vi "unwrap_phase_map_edge_detect_float.vi"(11 "u8_ar_dist_phasemap":dbl[][](array[numeric])=array1050x1050[1102500 elements]) -> (2 "df_ar_unwrapped_px_ar":dbl[][](array[numeric]), 3 "Refnum out":T3(plugin-control))   [LabVIEW 2011]
doc: "Takes a the warpped phase mapped as a pixel array and unwrappes it. Optional normalization from 0 to 255 for the pixel array output"
uses:
  <vilib>/vision/Measure.llb/Edge Options.ctl
  <vilib>/vision/Measure.llb/Edge Polarity.ctl
  global_vars.vi
  <vilib>/vision/NI_Vision_Development_Module.lvlib
panel:
  out "norm part":i16[](graph)
  out "unwrapped":dbl[](graph)
  out "norm factor":dbl
  out "offset":i16
  out "Intensity Graph 2":dbl[][](graph)
  out "Intensity Graph":dbl[][](graph)
  out "normalized array":u8[](array[numeric])
  out "normalized":u8[](graph)
  in  "Edge Options 3":T1={"Edge Polarity"=0, "Kernel Size"=3, "Width"=1, "Minimum Edge Strength"=250.0, "Interpolation Type"=enum."Bilinear Fixed", "Data Processing Method"=enum."Median"} {"Edge Polarity" items=["All Edges", "Rising Edges", "Falling Edges"]; "Minimum Edge Strength" format="%.2f"; "Width" step=2; "Kernel Size" step=2}
  out "start and end":i32[](array[numeric])
  out "edges":i16[](array[numeric])
  in  "stop":bool
  out "input":i16[](graph)
  in  "Edge Options 2":T1={"Edge Polarity"=0, "Kernel Size"=3, "Width"=1, "Minimum Edge Strength"=250.0, "Interpolation Type"=enum."Bilinear Fixed", "Data Processing Method"=enum."Median"} {"Edge Polarity" items=["All Edges", "Rising Edges", "Falling Edges"]; "Minimum Edge Strength" format="%.2f"; "Width" step=2; "Kernel Size" step=2}
  out "Waveform Graph 2":dbl[](graph)
  in  "index (row)":i32(slide) scale=0.0..1000.0
  out "Image":T3(plugin-control)
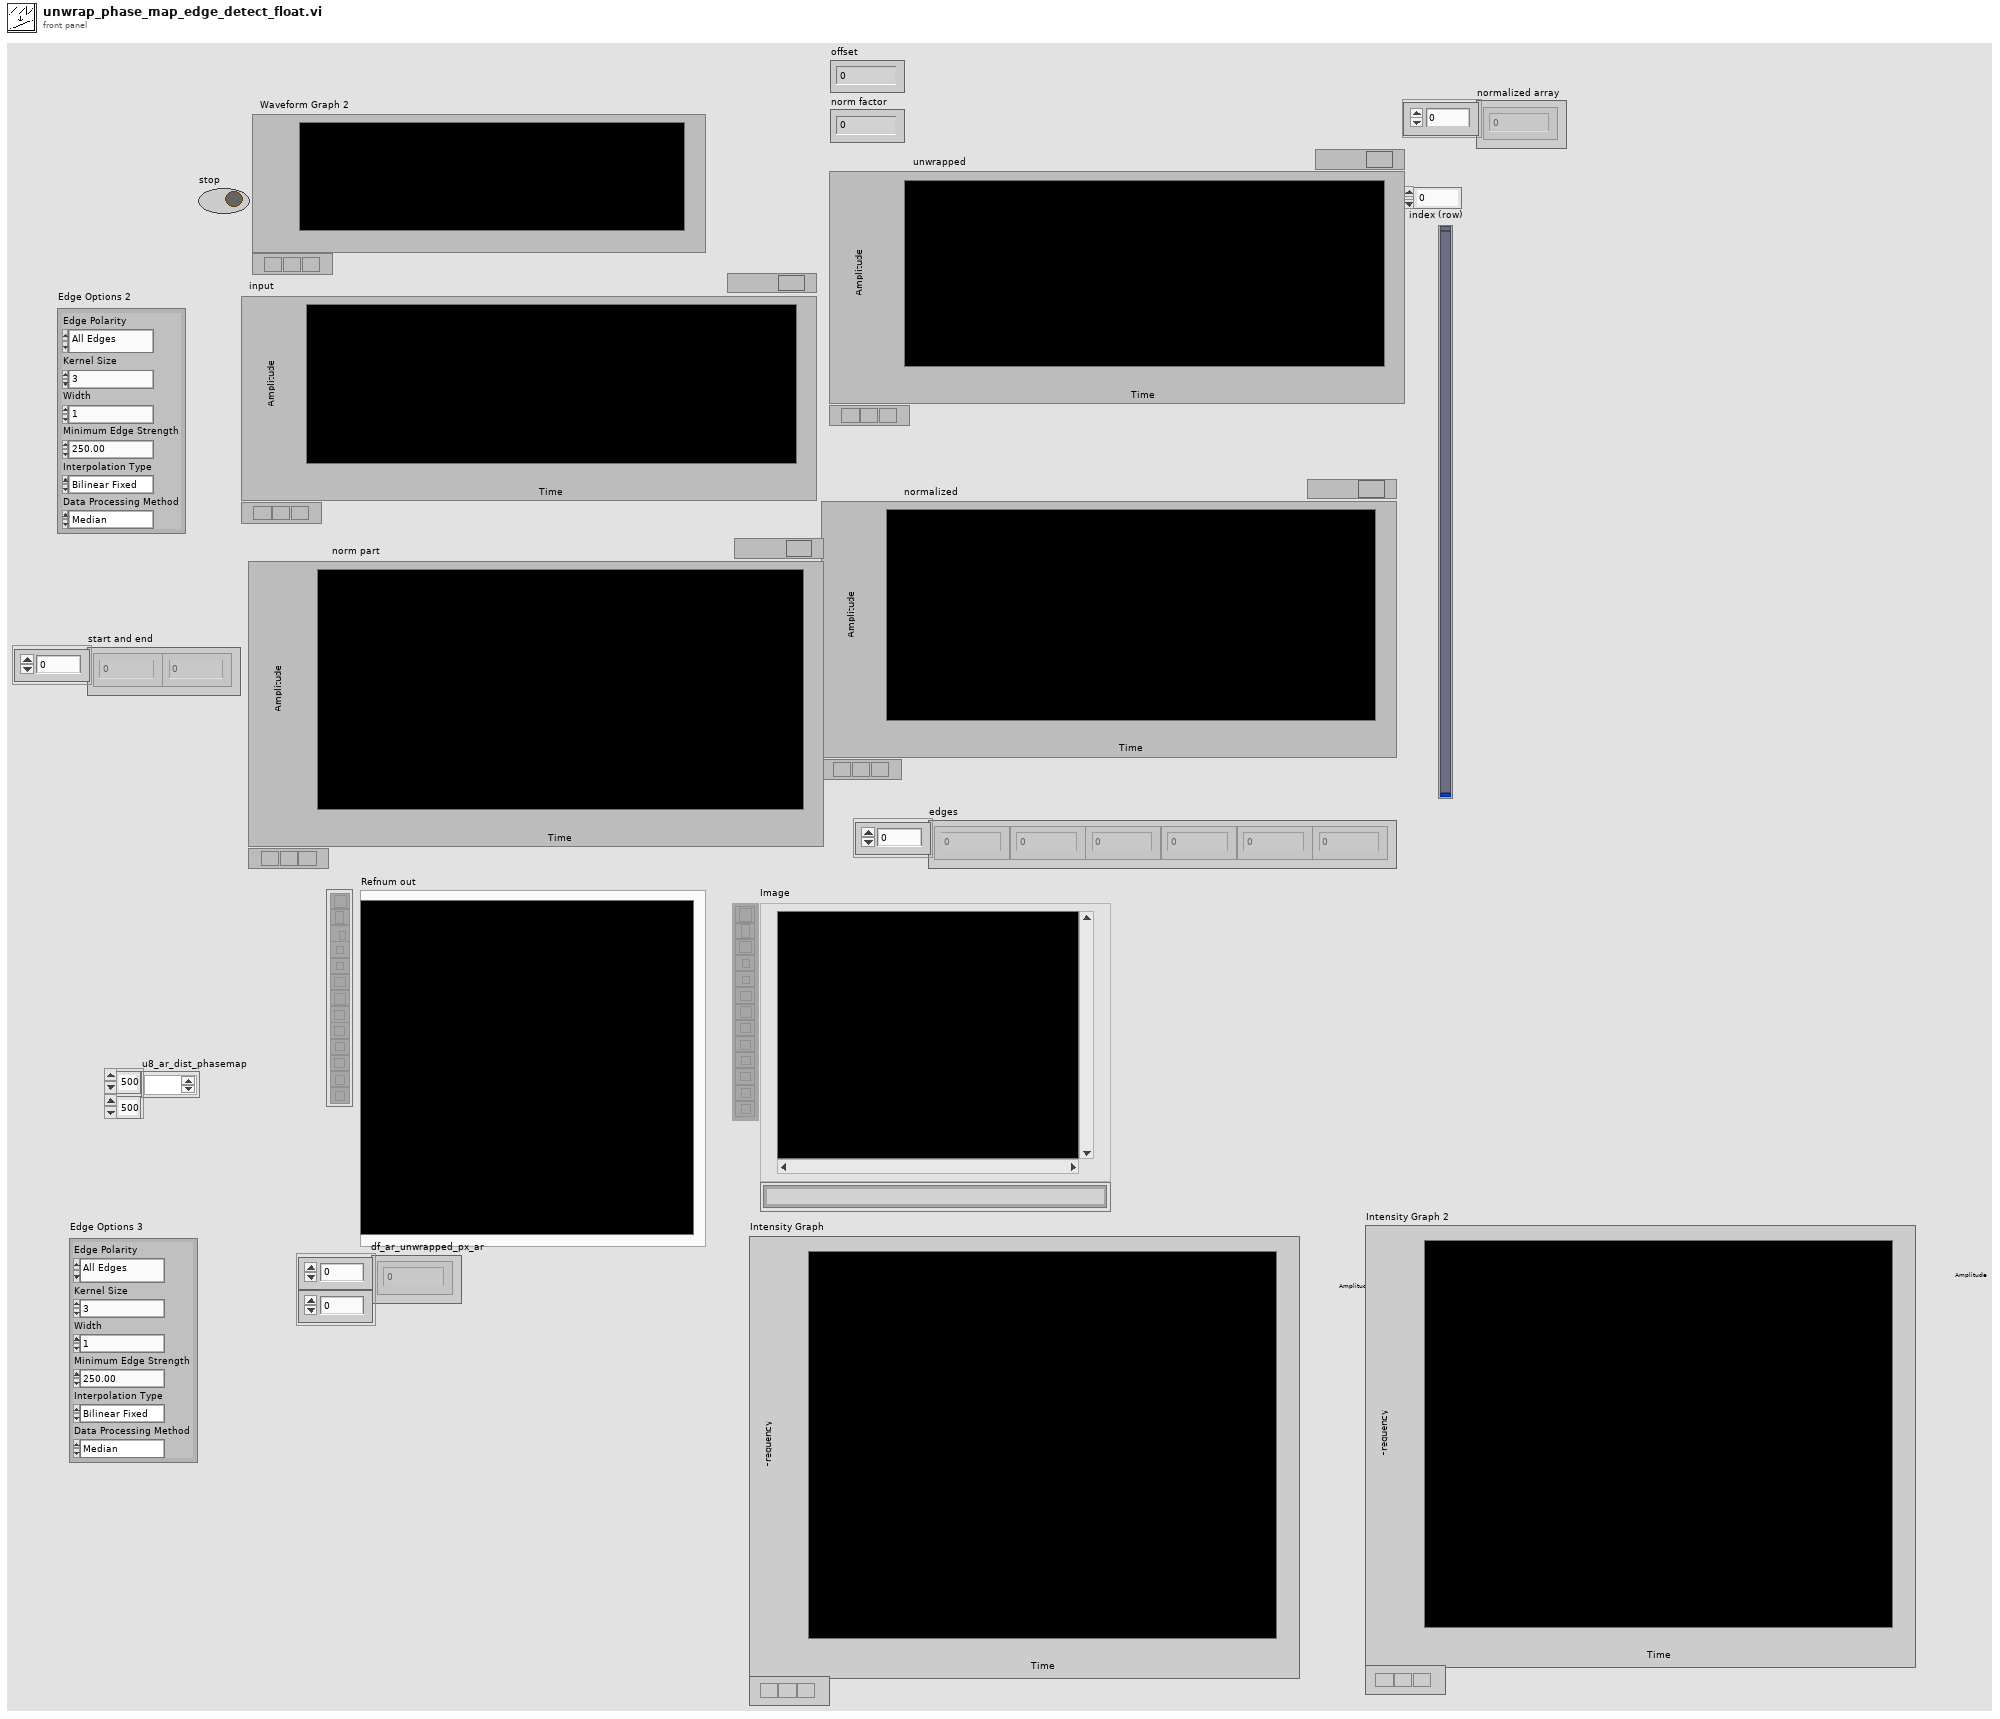
[diagram p1: front panel]
types:
  T1 = typedef "Edge Options.ctl" = cluster{"Edge Polarity":T2, "Kernel Size":u32, "Width":u32, "Minimum Edge Strength":sgl, "Interpolation Type":enum32{"Zero Order", "Bilinear", "Quadratic", "Cubic", "Bilinear Fixed"}, "Data Processing Method":enum32{"Average", "Median"}}
  T2 = typedef "Edge Polarity.ctl" = u32
  T3 = typedef "IMAQ Image.ctl" = refnum<image>
  T4 = typedef "Image Type" = u32
  T5 = typedef "IMAQ Line" = cluster{"Start X":i32, "Start Y":i32, "End X":i32, "End Y":i32}
  T6 = typedef "ROI Descriptor" = cluster{"Global Rectangle":i32[], "Contours":cluster{"ID":enum32{"External", "Internal"}, "Type":u32, "Coordinates":i32[]}[]}
  T7 = typedef "Edge New.ctl" = cluster{"Location (Pixel)":cluster{"X":sgl, "Y":sgl}, "Location (Real-World)":cluster{"X":sgl, "Y":sgl}, "Distance (Pixel)":dbl, "Distance (Real-World)":dbl, "Strength":dbl, "Noise":dbl, "Rising?":bool}
  T8 = enum16{"Get First Edge", "Get First + Last Edge", "Get All Edges", "Get Best Edge"}
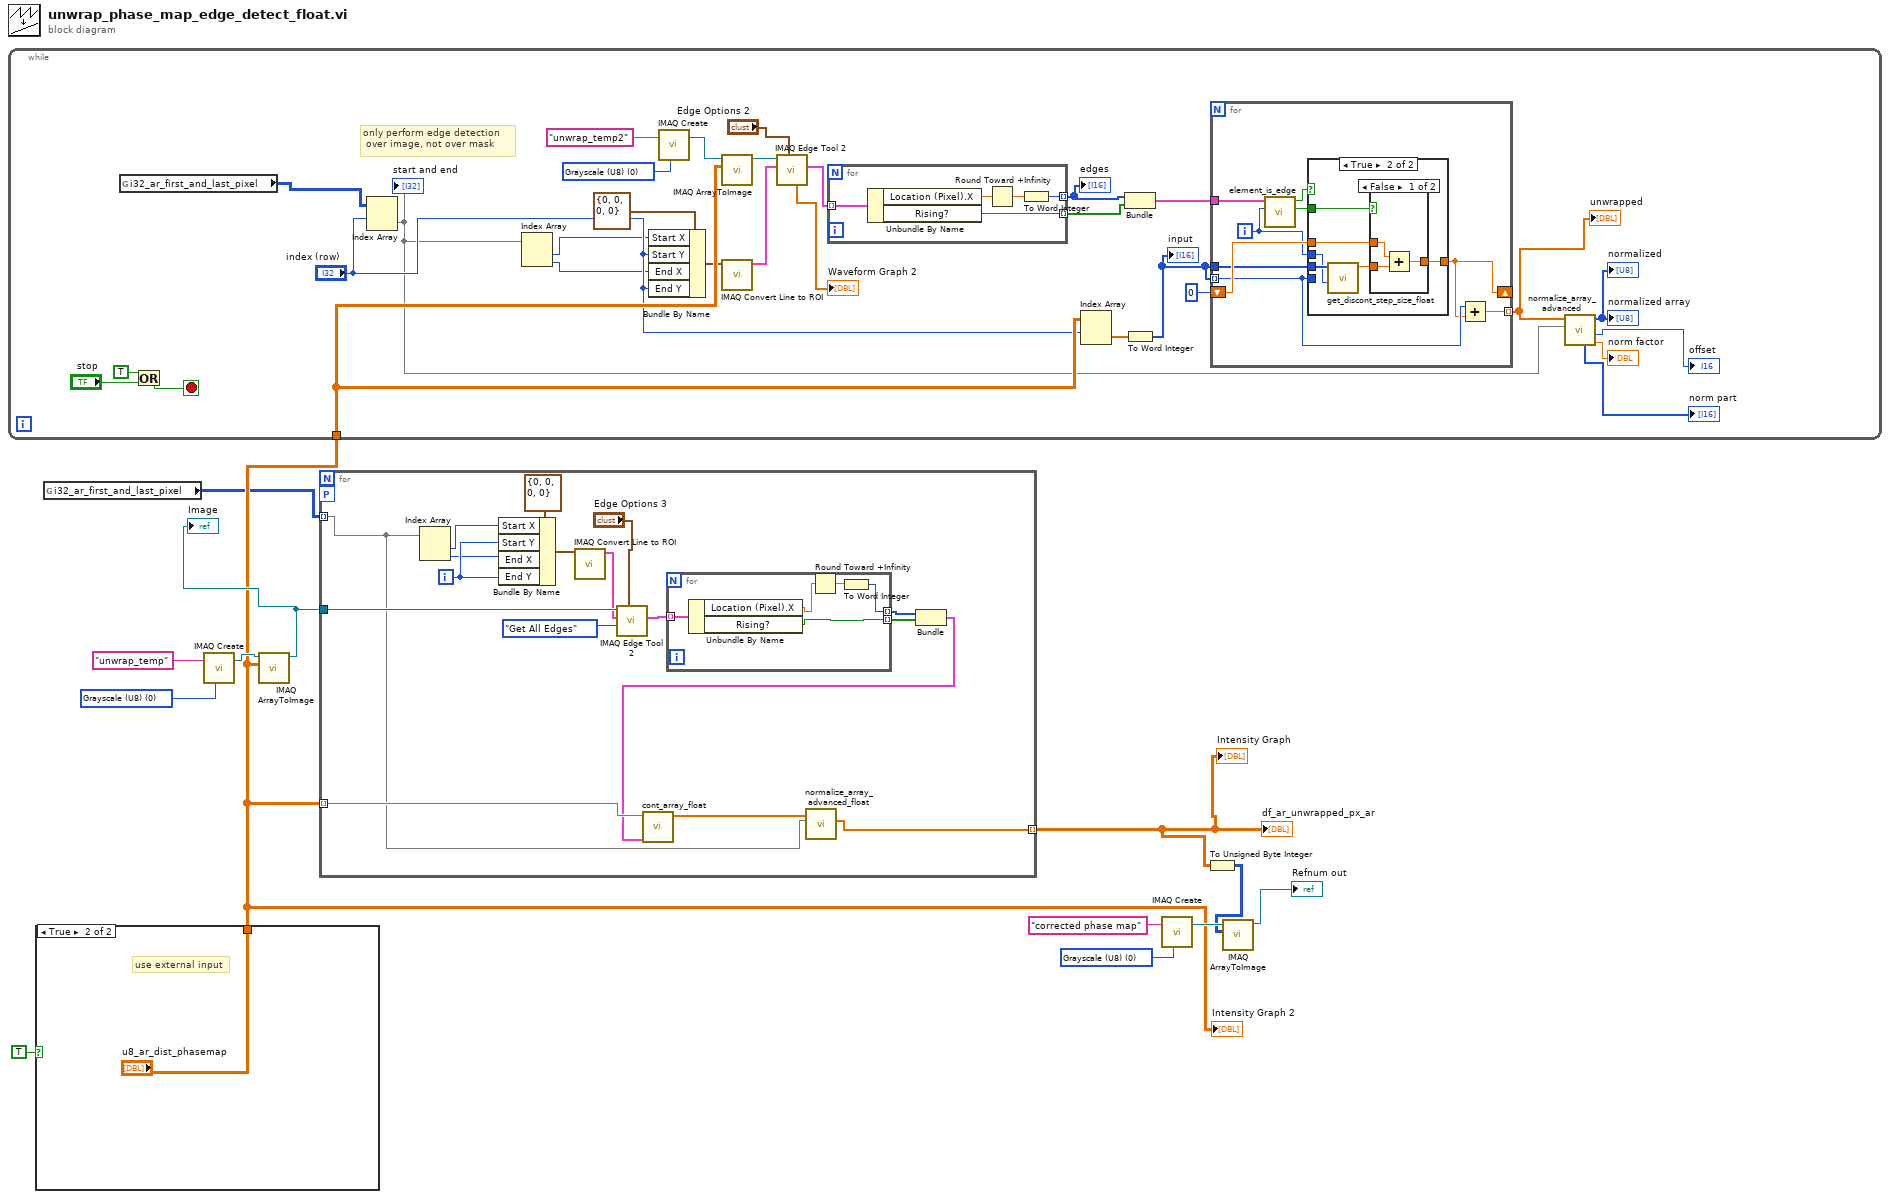
[diagram p0: block diagram]
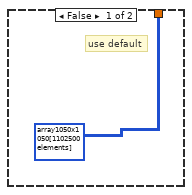
[diagram p2: hidden frame]
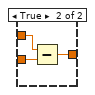
[diagram p4: hidden frame]
diagram:
  w7 = T4 0 items=["Grayscale (U8)", "Grayscale (I16)", "Grayscale (SGL)", "Complex (CSG)", "RGB (U32)", "HSL (U32)", "RGB (U64)", "Grayscale (U16)"] ("Image Type")
  w12 = T4 0 items=["Grayscale (U8)", "Grayscale (I16)", "Grayscale (SGL)", "Complex (CSG)", "RGB (U32)", "HSL (U32)", "RGB (U64)", "Grayscale (U16)"] ("Image Type")
  n1 = case shown="True" TRUE {
    tunnel: [u8[][] array1050x1050[1102500 elements] ("u8_ar_dist_phasemap") "u8_ar_dist_phasemap"] -> w4
    frame False {
      # "use default"
    }
    frame True {
      # "use external input"
    }
  }
  "Intensity Graph 2" <- w4
  n2 = while {
    tunnel: w4 -> [w39]
    stop <- w25 stop-if-true
    w42 = T4 0 items=["Grayscale (U8)", "Grayscale (I16)", "Grayscale (SGL)", "Complex (CSG)", "RGB (U32)", "HSL (U32)", "RGB (U64)", "Grayscale (U16)"] ("Image Type")
    # "only perform edge detection\n over image, not over mask"
    n3 = global read "global_vars.vi" "i32_ar_first_and_last_pixel"() -> (w20:i32[][])
    n4 = Or(x=TRUE, y="stop") -> (x .or. y?=w25:bool)
    n5 = Index Array(array=w20, index (row)="index (row)") -> (element=w22:i32[])  [unwired: 1 in]
    "start and end" <- w22
    n6 = Index Array(array=w22) -> (element #1=w27:i32, element #2=w26:i32)  [unwired: 2 in]
    n7 = Bundle By Name(cluster=T5 {"Start X"=0, "Start Y"=0, "End X"=0, "End Y"=0} ("Line 3"), "Start X"=w27, "Start Y"="index (row)", "End X"=w26, "End Y"="index (row)") -> (w37:T5)
    n8 = call "IMAQ Create"("Image Name"="unwrap_temp2", "Image Type"=w42) -> ("New Image"=w41:T3)  [unwired: 2 in, 2 out]
    n9 = call "IMAQ ArrayToImage"("Image Pixels (U8)"=w39, "Image"=w41) -> ("Image Out"=w40:T3)  [unwired: 8 in, 1 out]
    n10 = call "IMAQ Convert Line to ROI"("Line"=w37) -> ("ROI Descriptor"=w36:T6)  [unwired: 8 in, 1 out]
    n11 = call "IMAQ Edge Tool 2"("Edge Options"="Edge Options 2", "ROI Descriptor"=w36, "Image"=w40) -> ("Edge Information"=w30:T7[], "Gradient Values"=→"Waveform Graph 2":dbl[])  [unwired: 3 in, 4 out]
    n12 = for {
      tunnel: w30 -> [w50] mode=indexing
      tunnel: [w49] -> w33 mode=indexing
      tunnel: [w47] -> w29 mode=indexing
      n13 = Unbundle By Name(w50) -> ("Location (Pixel).X"=w46:sgl, "Rising?"=w49:bool)
      n14 = Round Toward +Infinity(x=w46) -> (ceil(x): smallest int >= x=w48:sgl)
      n15 = To Word Integer(number=w48) -> (16bit integer=w47:i16)
    }
    "edges" <- w29
    n16 = Index Array(array=w39, index (row)="index (row)") -> (element=w44:dbl[])  [unwired: 1 in]
    n17 = Bundle(w29, w33) -> (w32:cluster{i16[], bool[]})  [unwired: 1 in]
    n18 = To Word Integer(number=w44) -> (16bit integer=w31:i16[])
    "input" <- w31
    n19 = for {
      tunnel: w31 -> [w52]
      tunnel: w31 -> [w55] mode=indexing
      shift-right: [w51] -> _
      shift-left: i16 0 -> [w59]
      tunnel: [w58] -> w17 mode=indexing
      tunnel: w32 -> [w54]
      i -> [w53]
      n20 = call "element_is_edge.vi"("current element"=w53, "edge cluster"=w54) -> ("direction (rising/falling)"=w56:bool, "edge"=w57:bool)  [unwired: 8 in]
      n21 = case shown="True" w57 {
        tunnel: [w60 w65] -> w51
        tunnel: w59 -> [w60 w66]
        tunnel: w56 -> [_ w64]
        tunnel: w55 -> [_ _]
        tunnel: w53 -> [_ w62]
        tunnel: w52 -> [_ w63]
        frame False {
        }
        frame True {
          n22 = call "get_discont_step_size_float.vi"("current pixel (iteration)"=w62, "current row in image"=w63) -> ("step_size"=w61:dbl)  [unwired: 9 in]
          n23 = case shown="False" w64 {
            tunnel: w66 -> [w69 w72]
            tunnel: [w68 w71] -> w65
            tunnel: w61 -> [w67 w70]
            frame False {
              n24 = Add(x=w69, y=w67) -> (x+y=w68:dbl)
            }
            frame True {
              n25 = Subtract(x=w72, y=w70) -> (x-y=w71:dbl)
            }
          }
        }
      }
      n26 = Add(x=w55, y=w51) -> (x+y=w58:dbl)
    }
    "unwrapped" <- w17
    n27 = call "normalize_array_advanced.vi"("i32_ar_first_and_last_pixel"=w22, "unwrapped array"=w17) -> ("norm factor"=→"norm factor":dbl, "offset"=→"offset":i16, "normalized unwrapped array"=→"normalized" →"normalized array":u8[], "normalizing part"=→"norm part":i16[])  [unwired: 5 in, 1 out]
  }
  n28 = global read "global_vars.vi" "i32_ar_first_and_last_pixel"() -> (w3:i32[][])
  n29 = call "IMAQ Create"("Image Name"="unwrap_temp", "Image Type"=w12) -> ("New Image"=w11:T3)  [unwired: 2 in, 2 out]
  n30 = call "IMAQ ArrayToImage"("Image Pixels (U8)"=w4, "Image"=w11) -> ("Image Out"=w10:T3)  [unwired: 8 in, 1 out]
  "Image" <- w10
  n31 = for {
    tunnel: w4 -> [w89] mode=indexing
    tunnel: w10 -> [w87]
    workers-P: _ -> [_]
    tunnel: w3 -> [w74] mode=indexing
    tunnel: [w73] -> w2 mode=indexing
    i -> [w81]
    n32 = Index Array(array=w74) -> (element #1=w77:i32, element #2=w76:i32)  [unwired: 2 in]
    n33 = Bundle By Name(cluster=T5 {"Start X"=0, "Start Y"=0, "End X"=0, "End Y"=0} ("Line 2"), "Start X"=w77, "Start Y"=w81, "End X"=w76, "End Y"=w81) -> (w85:T5)
    n34 = call "IMAQ Convert Line to ROI"("Line"=w85) -> ("ROI Descriptor"=w84:T6)  [unwired: 8 in, 1 out]
    n35 = call "IMAQ Edge Tool 2"("Edge Options"="Edge Options 3", "Process"=T8."Get All Edges", "ROI Descriptor"=w84, "Image"=w87) -> ("Edge Information"=w83:T7[])  [unwired: 2 in, 5 out]
    n36 = for {
      tunnel: w83 -> [w94] mode=indexing
      tunnel: [w90] -> w80 mode=indexing
      tunnel: [w93] -> w79 mode=indexing
      n37 = Unbundle By Name(w94) -> ("Location (Pixel).X"=w91:sgl, "Rising?"=w93:bool)
      n38 = Round Toward +Infinity(x=w91) -> (ceil(x): smallest int >= x=w92:sgl)
      n39 = To Word Integer(number=w92) -> (16bit integer=w90:i16)
    }
    n40 = Bundle(w80, w79) -> (w82:cluster{i16[], bool[]})  [unwired: 1 in]
    n41 = call "cont_array_float.vi"("edge cluster"=w82, "u8_ar_phase map"=w89) -> ("Array"=w75:dbl[])  [unwired: 9 in]
    n42 = call "normalize_array_advanced_float.vi"("i32_ar_first_and_last_pixel"=w74, "unwrapped array"=w75) -> ("i16_normalized unwrapped array"=w73:dbl[])  [unwired: 5 in, 4 out]
  }
  "df_ar_unwrapped_px_ar" <- w2
  "Intensity Graph" <- w2
  n43 = call "IMAQ Create"("Image Name"="corrected phase map" ("corrected phase map"), "Image Type"=w7) -> ("New Image"=w6:T3)  [unwired: 2 in, 2 out]
  n44 = To Unsigned Byte Integer(number=w2) -> (unsigned 8bit integer=w1:u8[][])
  n45 = call "IMAQ ArrayToImage"("Image Pixels (U8)"=w1, "Image"=w6) -> ("Image Out"=→"Refnum out":T3)  [unwired: 8 in, 1 out]
